vi "syntax_parser.vi"(9 "Analyse":bool, 10 "Auto correction":bool, 11 "Chaîne IN":string) -> (1 "Chaîne analysée":string, 3 "Chaîne OUT":string)   [LabVIEW 2013]
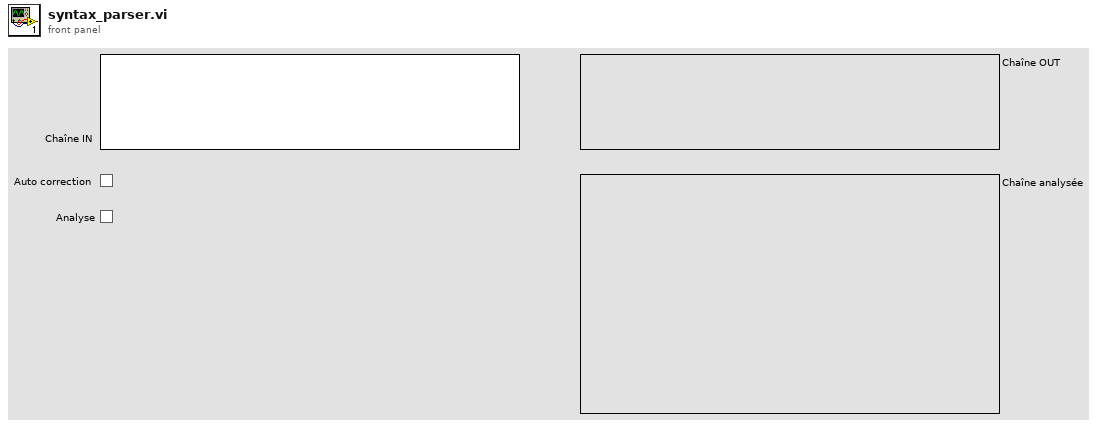
[diagram p1: front panel]
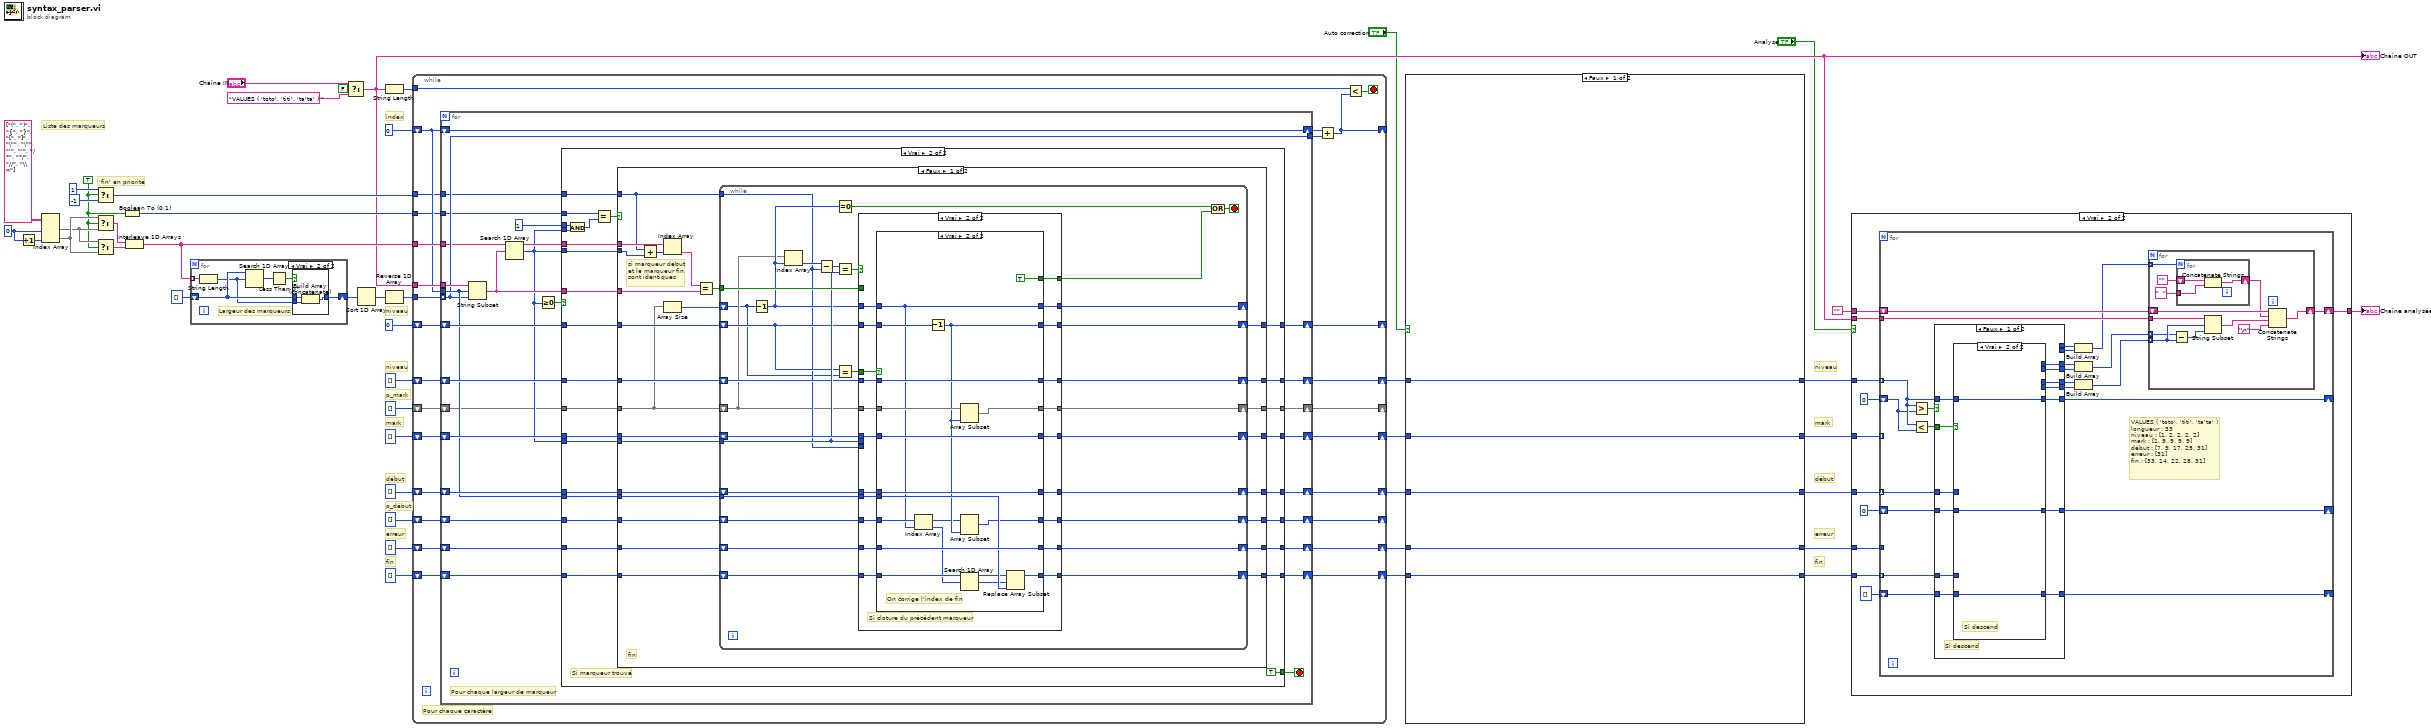
[diagram p0: block diagram]
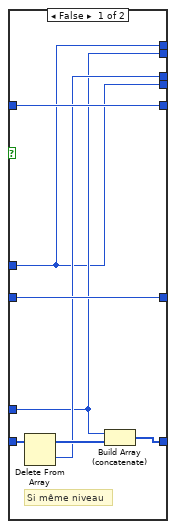
[diagram p4: hidden frame]
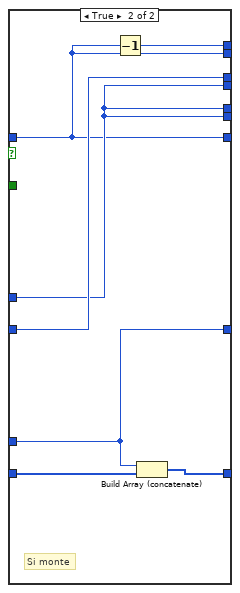
[diagram p5: hidden frame]
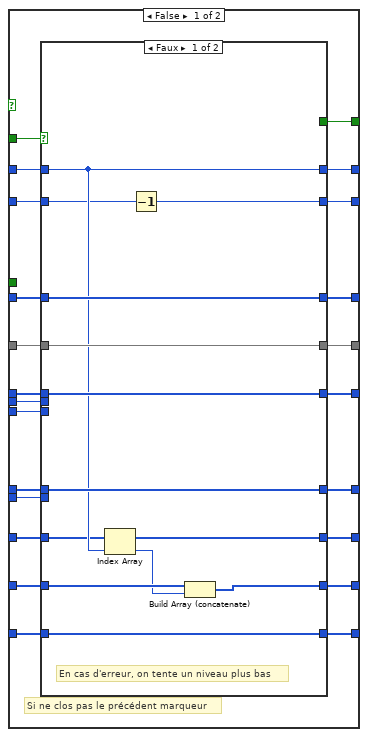
[diagram p7: hidden frame]
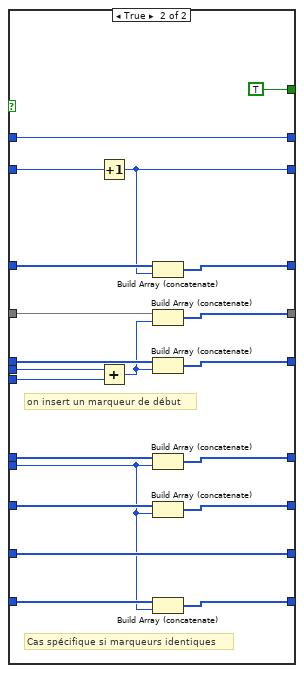
[diagram p8: hidden frame]
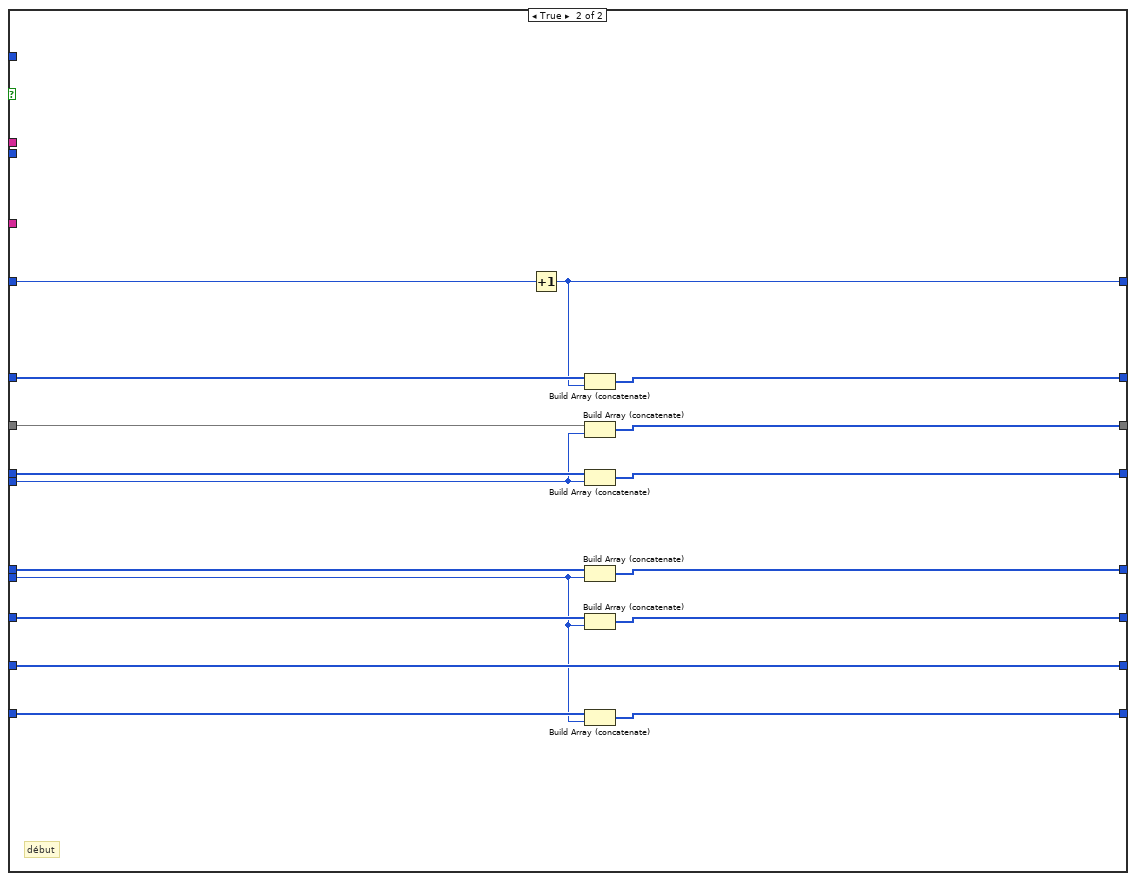
[diagram p10: hidden frame]
diagram:
  w20 = TRUE
  w43 = 0
  # "erreur"
  # "niveau"
  # "fin"
  # "début"
  # "mark"
  # "p_début"
  # "p_mark"
  # "'fin' en priorité"
  # "index"
  # "Liste des marqueurs"
  # "erreur"
  # "niveau"
  # "fin"
  # "début"
  # "mark"
  # "niveau"
  n1 = Increment(x=w43) -> (x+1=w44:i32)
  n2 = Index Array(array=string[][] [["(", ")"], ["{", "}"], ["[", "]"], ["\"", "\""], ["'", "'"], ["/*", "*/"], ["//", "\\n"]], index (col) #1=w43, index (col) #2=w44) -> (element #1=w24:string[], element #2=w25:string[])  [unwired: 2 in]
  n3 = Select(t=1, s=w20, f=-1) -> (s? t:f=w21:i32)
  n4 = Select(t=w25, s=w20, f=w24) -> (s? t:f=w27:string[])
  n5 = Select(t=w24, s=w20, f=w25) -> (s? t:f=w26:string[])
  n6 = Boolean To (0,1)(Boolean=w20) -> (0, 1=w19:i16)
  n7 = Interleave 1D Arrays(w27, w26) -> (w32:string[])
  n8 = for {
    tunnel: w32 -> [w51] mode=indexing
    shift-right: [w48] -> w35
    shift-left: i32[] [] -> [w47]
    # "Largeur des marqueurs"
    n9 = String Length(string=w51) -> (length=w46:i32)
    n10 = Search 1D Array(1D array=w47, element=w46) -> (index of element=w50:i32)  [unwired: 1 in]
    n11 = Less Than 0?(x=w50) -> (x < 0?=w49:bool)
    n12 = case shown="Vrai" w49 {
      tunnel: [w52 w54] -> w48
      tunnel: w47 -> [w52 w55]
      tunnel: w46 -> [_ w53]
      frame False {
      }
      frame True {
        n13 = Build Array (concatenate)(w55, w53) -> (w54:i32[])
      }
    }
  }
  n14 = Select(t="Chaîne IN", s=FALSE, f="VALUES ( 'toto', 'titi', 'ta'ta' ) ") -> (s? t:f=w15:string)
  "Chaîne OUT" <- w15
  n15 = Sort 1D Array(array=w35) -> (sorted array=w34:i32[])
  n16 = String Length(string=w15) -> (length=w30:i32)
  n17 = Reverse 1D Array(array=w34) -> (reversed array=w33:i32[])
  n18 = while {
    tunnel: w15 -> [w82]
    shift-right: [w68] -> _
    shift-left: 0 -> [w74]
    shift-right: [w69] -> w10
    shift-left: i32[] [] -> [w75]
    shift-right: [w70] -> w9
    shift-left: i32[] [] -> [w76]
    shift-right: [w71] -> w8
    shift-left: i32[] [] -> [w77]
    shift-right: [w72] -> w11
    shift-left: i32[] [] -> [w78]
    shift-right: [w73] -> w1
    shift-left: i32[] [] -> [w79]
    tunnel: w33 -> [w81]
    tunnel: w32 -> [w80]
    shift-right: [w63] -> _
    shift-left: 0 -> [w67]
    tunnel: w30 -> [w62]
    tunnel: w21 -> [w61]
    tunnel: w19 -> [w60]
    shift-right: [w59] -> _
    shift-left: i32[] [] -> [w58]
    shift-right: [w57] -> _
    shift-left: i32[] [] -> [w56]
    stop <- w64 stop-if-true
    # "Pour chaque caractère"
    n19 = for {
      tunnel: w82 -> [w110]
      tunnel: w67 -> [w95]
      tunnel: w81 -> [w93] mode=indexing
      tunnel: w80 -> [w92]
      shift-right: [w98] -> w68
      shift-left: w74 -> [w97]
      shift-right: [w100] -> w69
      shift-left: w75 -> [w99]
      shift-right: [w102] -> w70
      shift-left: w76 -> [w101]
      shift-right: [w104] -> w71
      shift-left: w77 -> [w103]
      shift-right: [w106] -> w72
      shift-left: w78 -> [w105]
      shift-right: [w108] -> w73
      shift-left: w79 -> [w107]
      shift-right: [w94] -> w65
      shift-left: w67 -> [w94]
      tunnel: [w93] -> w66
      tunnel: w61 -> [w90]
      tunnel: w60 -> [w87]
      shift-right: [w85] -> w59
      shift-left: w58 -> [w86]
      shift-right: [w83] -> w57
      shift-left: w56 -> [w84]
      stop <- w96 stop-if-true
      # "Pour chaque largeur de marqueur"
      n20 = String Subset(string=w110, offset (0)=w95, length (rest)=w93) -> (substring=w91:string)
      n21 = Search 1D Array(1D array=w92, element=w91) -> (index of element=w89:i32)  [unwired: 1 in]
      n22 = Greater Or Equal To 0?(x=w89) -> (x >= 0?=w109:bool)
      n23 = case shown="Vrai" w109 {
        tunnel: [w118 w136] -> w108
        tunnel: w107 -> [w118 w137]
        tunnel: [w117 w138] -> w106
        tunnel: w105 -> [w117 w139]
        tunnel: [w116 w134] -> w104
        tunnel: w103 -> [w116 w135]
        tunnel: [w115 w132] -> w102
        tunnel: w101 -> [w115 w133]
        tunnel: [w114 w141] -> w100
        tunnel: w99 -> [w114 w142]
        tunnel: [w113 w143] -> w98
        tunnel: w97 -> [w113 w144]
        tunnel: 1 -> [_ w146]
        tunnel: [_ TRUE] -> w96
        tunnel: w89 -> [_ w145]
        tunnel: w89 -> [_ w140]
        tunnel: w95 -> [_ w131]
        tunnel: w92 -> [_ w129]
        tunnel: w89 -> [_ w128]
        tunnel: w91 -> [_ w127]
        tunnel: w90 -> [_ w126]
        tunnel: w87 -> [_ w123]
        tunnel: [w112 w122] -> w85
        tunnel: w86 -> [w112 w121]
        tunnel: [w111 w120] -> w83
        tunnel: w84 -> [w111 w119]
        frame False {
          # "Si pas de marqueur trouvé"
        }
        frame True {
          # "Si marqueur trouvé"
          n24 = And(x=w146, y=w145) -> (x .and. y?=w125:i32)
          n25 = Equal?(x=w123, y=w125) -> (x = y?=w124:bool)
          n26 = case shown="Faux" w124 {
            tunnel: w144 -> [w154 w322]
            tunnel: [w172 w310] -> w143
            tunnel: w142 -> [w153 w321]
            tunnel: [w164 w320] -> w141
            tunnel: w140 -> [w155 w309]
            tunnel: w139 -> [w160 w319]
            tunnel: [w165 w318] -> w138
            tunnel: w137 -> [w158 w317]
            tunnel: [w162 w317] -> w136
            tunnel: w135 -> [w157 w314]
            tunnel: [w161 w313] -> w134
            tunnel: w133 -> [w159 w316]
            tunnel: [w163 w315] -> w132
            tunnel: w131 -> [w151 w306]
            tunnel: w129 -> [w171 _]
            tunnel: w128 -> [w169 _]
            tunnel: w127 -> [w168 _]
            tunnel: w126 -> [w156 _]
            tunnel: w121 -> [w147 w311]
            tunnel: [w150 w312] -> w122
            tunnel: w119 -> [w149 w308]
            tunnel: [w148 w307] -> w120
            frame False {
              # "si marqueur début\net le marqueur fin\nsont identiques"
              # "fin"
              n27 = Add(x=w156, y=w169) -> (x+y=w170:i32)
              n28 = Index Array(array=w171, index=w170) -> (element=w167:string)
              n29 = Array Size(array=w147) -> (size(s)=w152:i32)
              n30 = Equal?(x=w167, y=w168) -> (x = y?=w166:bool)
              n31 = while {
                shift-right: [w192] -> w172
                shift-left: w154 -> [w180]
                shift-right: [w193] -> w165
                shift-left: w160 -> [w181]
                shift-right: [w194] -> w164
                shift-left: w153 -> [w198]
                shift-right: [w195] -> w163
                shift-left: w159 -> [w199]
                shift-right: [w196] -> w162
                shift-left: w158 -> [w200]
                shift-right: [w197] -> w161
                shift-left: w157 -> [w201]
                tunnel: w166 -> [w187]
                tunnel: w156 -> [w177]
                tunnel: w155 -> [w183]
                shift-right: [w191] -> _
                shift-left: w152 -> [w173]
                tunnel: w151 -> [w185]
                shift-right: [w184] -> w150
                shift-left: w147 -> [w174]
                shift-right: [w176] -> w148
                shift-left: w149 -> [w175]
                stop <- w190 stop-if-true
                n32 = Decrement(x=w173) -> (x-1=w182:i32)
                n33 = Index Array(array=w174, index=w182) -> (element=w178:i32)
                n34 = Subtract(x=w178, y=w177) -> (x-y=w202:i32)
                n35 = Equal To 0?(x=w182) -> (x = 0?=w189:bool)
                n36 = Equal?(x=w202, y=w183) -> (x = y?=w188:bool)
                n37 = Equal?(x=w180, y=w173) -> (x = y?=w179:bool)
                n38 = case shown="Vrai" w188 {
                  tunnel: [w211 w270] -> w197
                  tunnel: w201 -> [w218 w273]
                  tunnel: [w216 w269] -> w196
                  tunnel: w200 -> [w219 w274]
                  tunnel: [w212 w268] -> w195
                  tunnel: w199 -> [w220 w275]
                  tunnel: [w217 w267] -> w194
                  tunnel: w198 -> [w221 w276]
                  tunnel: [w213 w266] -> w193
                  tunnel: w181 -> [w222 w272]
                  tunnel: [w214 w264] -> w192
                  tunnel: w180 -> [w223 w279]
                  tunnel: [w215 w263] -> w191
                  tunnel: w182 -> [w224 w271]
                  tunnel: w187 -> [w225 _]
                  tunnel: [w210 w262] -> w186
                  tunnel: w185 -> [w209 w261]
                  tunnel: w174 -> [w208 w278]
                  tunnel: [w207 w265] -> w184
                  tunnel: w183 -> [w206 _]
                  tunnel: w179 -> [_ w277]
                  tunnel: w177 -> [w205 _]
                  tunnel: [w204 w260] -> w176
                  tunnel: w175 -> [w203 w259]
                  frame False {
                    # "Si ne clos pas le précédent marqueur"
                    n39 = case shown="Faux" w225 {
                      tunnel: [w229 w253] -> w215
                      tunnel: w224 -> [w229 w253]
                      tunnel: [w226 w244] -> w214
                      tunnel: w223 -> [w227 w254]
                      tunnel: [w237 w252] -> w213
                      tunnel: w222 -> [w237 w255]
                      tunnel: [w236 w251] -> w217
                      tunnel: w221 -> [w236 w256]
                      tunnel: [w230 w250] -> w212
                      tunnel: w220 -> [w230 w257]
                      tunnel: [w232 w249] -> w216
                      tunnel: w219 -> [w233 w249]
                      tunnel: [w235 w248] -> w211
                      tunnel: w218 -> [w235 w258]
                      tunnel: [_ TRUE] -> w210
                      tunnel: w209 -> [_ w239]
                      tunnel: [w234 w246] -> w207
                      tunnel: w208 -> [w234 w245]
                      tunnel: w206 -> [_ w243]
                      tunnel: w205 -> [_ w242]
                      tunnel: [w228 w240] -> w204
                      tunnel: w203 -> [w228 w241]
                      frame False {
                        # "En cas d'erreur, on tente un niveau plus bas"
                        n40 = Index Array(array=w228, index=w229) -> (element=w231:i32)
                        n41 = Decrement(x=w227) -> (x-1=w226:i32)
                        n42 = Build Array (concatenate)(w233, w231) -> (w232:i32[])
                      }
                      frame True {
                        # "on insert un marqueur de début"
                        # "Cas spécifique si marqueurs identiques"
                        n43 = Increment(x=w254) -> (x+1=w244:i32)
                        n44 = Add(x=w243, y=w242) -> (x+y=w238:i32)
                        n45 = Build Array (concatenate)(w255, w244) -> (w252:i32[])
                        n46 = Build Array (concatenate)(w245, w238) -> (w246:i32[])
                        n47 = Build Array (concatenate)(w256, w238) -> (w251:i32[])
                        n48 = Build Array (concatenate)(w257, w239) -> (w250:i32[])
                        n49 = Build Array (concatenate)(w241, w239) -> (w240:i32[])
                        n50 = Build Array (concatenate)(w258, w239) -> (w248:i32[])
                      }
                    }
                  }
                  frame True {
                    # "Si cloture du précédent marqueur"
                    n51 = case shown="Vrai" w277 {
                      tunnel: w279 -> [w283 w305]
                      tunnel: w278 -> [w284 w304]
                      tunnel: [w284 w303] -> w265
                      tunnel: [w283 w294] -> w264
                      tunnel: [w286 w302] -> w267
                      tunnel: w276 -> [w286 w302]
                      tunnel: [w288 w301] -> w268
                      tunnel: w275 -> [w288 w301]
                      tunnel: [w281 w300] -> w269
                      tunnel: w274 -> [w281 w300]
                      tunnel: [w287 w297] -> w270
                      tunnel: w273 -> [w287 w291]
                      tunnel: [w285 w299] -> w266
                      tunnel: w272 -> [w285 w299]
                      tunnel: [w282 w292] -> w263
                      tunnel: w271 -> [w282 w292]
                      tunnel: [_ TRUE] -> w262
                      tunnel: w261 -> [_ w296]
                      tunnel: [w280 w295] -> w260
                      tunnel: w259 -> [w280 w293]
                      frame False {
                        # "Parcours la liste à l'envers (devrait utiliser la pile)"
                      }
                      frame True {
                        # "On corrige l'index de fin"
                        n52 = Index Array(array=w293, index=w292) -> (element=w289:i32)
                        n53 = Decrement(x=w305) -> (x-1=w294:i32)
                        n54 = Array Subset(array=w304, length=w294) -> (w303:i32[])  [unwired: 1 in]
                        n55 = Array Subset(array=w293, length=w294) -> (w295:i32[])  [unwired: 1 in]
                        n56 = Search 1D Array(1D array=w291, element=w289) -> (index of element=w290:i32)  [unwired: 1 in]
                        n57 = Replace Array Subset(array=w291, new element=w296, index=w290) -> (w297:i32[])
                      }
                    }
                  }
                }
                n58 = Compound Arithmetic op=OR(w189, w186) -> (w190:bool)
              }
            }
            frame True {
              # "début"
              n59 = Increment(x=w322) -> (x+1=w310:i32)
              n60 = Build Array (concatenate)(w319, w310) -> (w318:i32[])
              n61 = Build Array (concatenate)(w311, w309) -> (w312:i32[])
              n62 = Build Array (concatenate)(w321, w309) -> (w320:i32[])
              n63 = Build Array (concatenate)(w316, w306) -> (w315:i32[])
              n64 = Build Array (concatenate)(w308, w306) -> (w307:i32[])
              n65 = Build Array (concatenate)(w314, w306) -> (w313:i32[])
            }
          }
        }
      }
    }
    n66 = Add(x=w65, y=w66) -> (x+y=w63:i32)
    n67 = Less?(x=w62, y=w63) -> (x < y?=w64:bool)
  }
  n68 = case shown="Faux" "Auto correction" {
    tunnel: [w327 w332] -> w7
    tunnel: w11 -> [w327 w332]
    tunnel: [w326 w331] -> w6
    tunnel: w10 -> [w326 w331]
    tunnel: [w325 w330] -> w5
    tunnel: w9 -> [w325 w330]
    tunnel: [w324 w329] -> w4
    tunnel: w8 -> [w324 w329]
    tunnel: [w323 w328] -> w2
    tunnel: w1 -> [w323 w328]
    frame False {
    }
    frame True {
    }
  }
  n69 = case shown="Vrai" "Analyse" {
    tunnel: w7 -> [_ w344]
    tunnel: w6 -> [_ w343]
    tunnel: w5 -> [_ w342]
    tunnel: w4 -> [_ w341]
    tunnel: w15 -> [_ w340]
    tunnel: [w333 w339] -> w14
    tunnel: "" -> [w333 w338]
    tunnel: w2 -> [_ w334]
    frame False {
    }
    frame True {
      n70 = for {
        tunnel: w344 -> [w350] mode=indexing
        tunnel: w343 -> [_] mode=indexing
        tunnel: w342 -> [w360] mode=indexing
        tunnel: w341 -> [w362] mode=indexing
        tunnel: w340 -> [w367]
        shift-right: [w365] -> w339
        shift-left: w338 -> [w366]
        shift-right: [w358] -> _
        shift-left: i32[] [] -> [w359]
        shift-right: [w351] -> _
        shift-left: 0 -> [w349]
        shift-right: [w361] -> _
        shift-left: 0 -> [w363]
        tunnel: w334 -> [_]
        # "VALUES ( 'toto', 'titi', 'ta'ta' ) \nlongueur : 33\nniveau : [1, 2, 2, 2, 2]\nmark : [1, 9, 9, 9, 9]\ndébut : [7, 9, 17, 25, 31]\nerreur : [31]\nfin : [33, 14, 22, 28, 31]"
        n71 = Greater?(x=w350, y=w349) -> (0:w364:bool)
        n72 = Less?(x=w350, y=w349) -> (x < y?=w348:bool)
        n73 = case shown="Faux" w364 {
          tunnel: w363 -> [w391 w412]
          tunnel: w362 -> [w385 w408]
          tunnel: [w392 w408] -> w361
          tunnel: w360 -> [w387 w411]
          tunnel: w359 -> [w389 w407]
          tunnel: [w390 w413] -> w358
          tunnel: [w388 w412] -> w355
          tunnel: [w386 w411] -> w354
          tunnel: [w384 w411] -> w353
          tunnel: [w383 w411] -> w352
          tunnel: w350 -> [w393 w409]
          tunnel: [w394 w409] -> w351
          tunnel: w348 -> [w395 _]
          tunnel: [_ w409] -> w346
          tunnel: [_ w410] -> w345
          frame False {
            # "Si descend"
            n74 = case shown="Vrai" w395 {
              tunnel: [w403 w404] -> w394
              tunnel: w393 -> [w403 w404]
              tunnel: [w402 w405] -> w392
              tunnel: w391 -> [w402 w405]
              tunnel: [w400 w406] -> w390
              tunnel: w389 -> [w401 w406]
              tunnel: [w396 _] -> w388
              tunnel: w387 -> [w396 _]
              tunnel: [w397 _] -> w386
              tunnel: w385 -> [w397 _]
              tunnel: [w398 _] -> w384
              tunnel: [w396 _] -> w383
              frame False {
                # "Si même niveau"
                n75 = Delete From Array(array=w401) -> (deleted portion=w398:i32, array with subset deleted=w399:i32[])  [unwired: 2 in]
                n76 = Build Array (concatenate)(w397, w399) -> (w400:i32[])
              }
              frame True {
                # "Si descend"
              }
            }
          }
          frame True {
            # "Si monte"
            n77 = Decrement(x=w409) -> (x-1=w410:i32)
            n78 = Build Array (concatenate)(w408, w407) -> (w413:i32[])
          }
        }
        n79 = Build Array(w345, w346) -> (w347:i32[])
        n80 = Build Array(w355, w354) -> (w357:i32[])
        n81 = Build Array(w353, w352) -> (w356:i32[])
        n82 = for {
          tunnel: w367 -> [w379]
          tunnel: w356 -> [w370] mode=indexing
          tunnel: w357 -> [w369] mode=indexing
          tunnel: w347 -> [w368] mode=indexing
          shift-right: [w377] -> w365
          shift-left: w366 -> [w378]
          n83 = Subtract(x=w369, y=w370) -> (x-y=w376:i32)
          n84 = for {
            N: w368 -> [_]
            tunnel: "  " -> [w381]
            shift-right: [w380] -> w371
            shift-left: "" -> [w382]
            n85 = Concatenate Strings(w382, w381) -> (w380:string)
          }
          n86 = String Subset(string=w379, offset (0)=w370, length (rest)=w376) -> (substring=w374:string)
          n87 = Concatenate Strings(w378, w371, w374, "\n") -> (w377:string)
        }
      }
    }
  }
  "Chaîne analysée" <- w14
